vi "FormatErrorToString.vi"(10 "error in":errorcluster, 11 "ErrorToLog":errorcluster) -> (2 "error out":errorcluster, 3 "ErrorString":string)   [LabVIEW 2017, in "Server.lvlib" / "ErrorLogger.lvlib"]
doc: "This SubVI generates a formatted String from the ErrorToLog-Input. It also contains a current Timestamp.\nExample-String:\n01.12.2017 12:20:05 Code: 12345 Source: This is a Test Error."
uses:
  ErrorLogger.lvlib
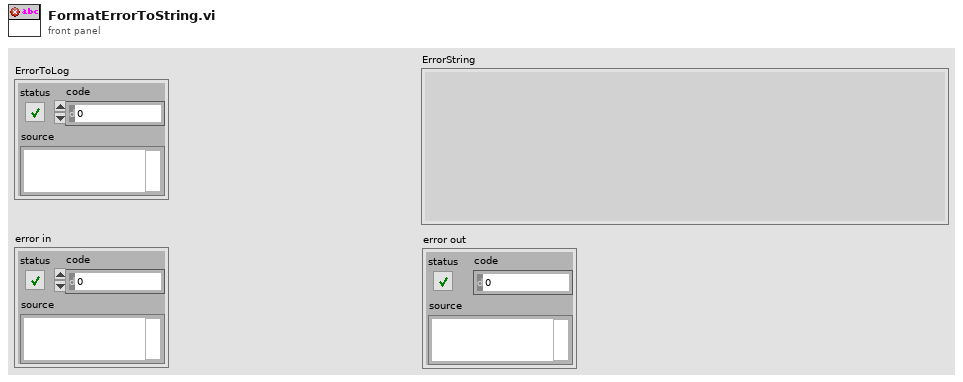
[diagram p1: front panel]
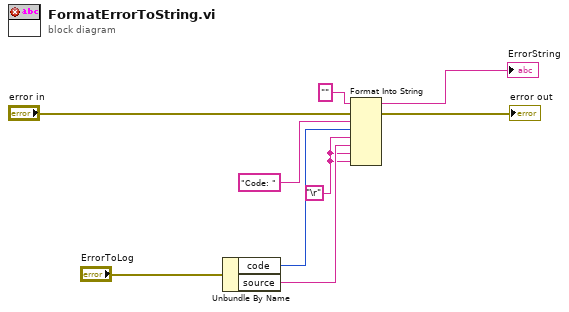
[diagram p0: block diagram]
diagram:
  w1 = "\r"
  n1 = Unbundle By Name("ErrorToLog") -> ("code"=w5:i32, "source"=w2:string)
  n2 = Format Into String(initial string="", error in="error in", "Code: " ("initial string"), w5, w1, w2, w1, w1) -> (resulting string=→"ErrorString":string, error out=→"error out":errorcluster)  [unwired: 1 in]
